vi "Incremental_Sums.vi"(11 "Array":dbl[](array[numeric])) -> (0 "output array":dbl[](array[numeric]))   [LabVIEW 2019]
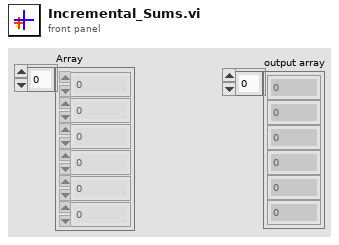
[diagram p1: front panel]
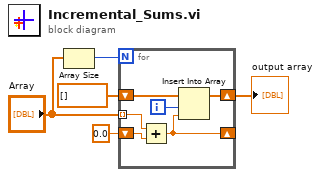
[diagram p0: block diagram]
diagram:
  n1 = Array Size(array="Array") -> (size(s)=w4:i32)
  n2 = for {
    N: w4 -> [_]
    shift-right: [w9] -> _
    shift-left: 0.0 -> [w11]
    tunnel: "Array" -> [w10] mode=indexing
    shift-right: [w6] -> w2
    shift-left: dbl[] [] -> [w7]
    i -> [w8]
    n3 = Add(x=w10, y=w11) -> (x+y=w9:dbl)
    n4 = Insert Into Array(array=w7, index=w8, new element=w9) -> (w6:dbl[])
  }
  "output array" <- w2
